vi "BucleFor_Arrays.vi"() -> ()   [LabVIEW 2020]
panel:
  out "number: 0 to 1":dbl
  out "Array 3":dbl[](array[numeric])
  out "i":i32
  in  "Array 2":dbl[][](array[numeric])
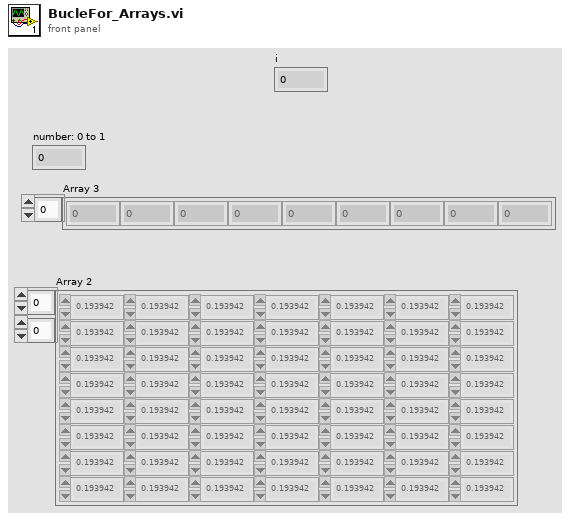
[diagram p1: front panel]
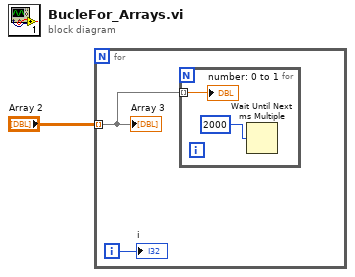
[diagram p0: block diagram]
diagram:
  n1 = for {
    tunnel: "Array 2" -> [w2] mode=indexing
    i -> [w3]
    n2 = for {
      tunnel: w2 -> [w5] mode=indexing
      n3 = Wait Until Next ms Multiple(millisecond multiple=u32 2000) -> ()  [unwired: 1 out]
      "number: 0 to 1" <- w5
    }
    "i" <- w3
    "Array 3" <- w2
  }
